vi "Read Enabled Channel Values.vi"(8 "error in (no error)":errorcluster, 11 "Multi Parser in":refnum<class "Multi Sentence Parser.lvclass">) -> (0 "error out":errorcluster, 2 "Enabled Values":dbl[](array[numeric]), 3 "Multi Parser out":refnum<class "Multi Sentence Parser.lvclass">)   [LabVIEW 2024, in "Multi Sentence Parser.lvclass"]
doc: "Multi Sentence Parser.lvclass:Read Enabled Channel Values.vi\n\nThis VI returns the data values of all the channels that are enabled for the Multi Sentence Parser class.\n\nInstrument Communication Module Version 1.0\nOctober, 2018 Original Code Consulting David Thomson\n www.originalcode.com"
uses:
  Multi Sentence Parser.lvclass
  Multi Sentence Parser.lvclass/Multi Sentence Parser.ctl
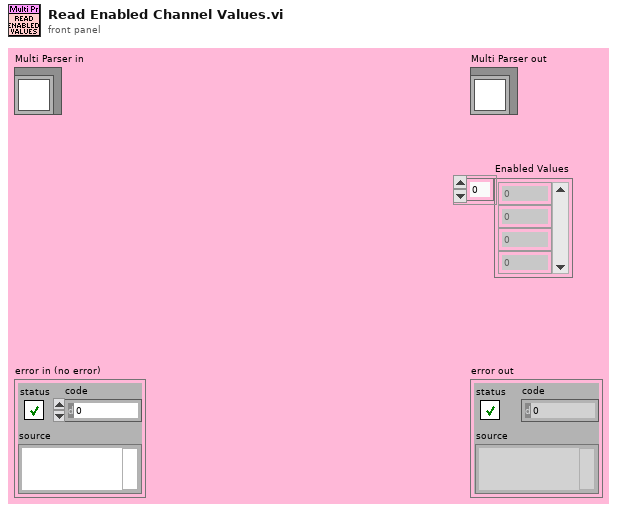
[diagram p1: front panel]
types:
  T1 = cluster{"Sentence ID":string, "Format String":string, "Channels":string[], "Enabled":bool[], "Ignore Missing Sentences?":bool}[]
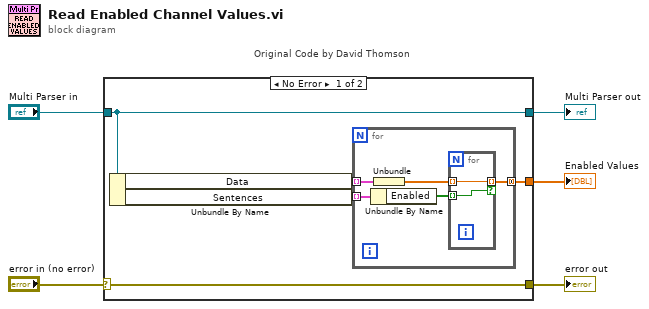
[diagram p0: block diagram]
diagram:
  n1 = case "Original Code by David Thomson" shown="No Error" "error in (no error)" {
    selector: "error in (no error)" -> [w10 w18]
    tunnel: [w10 w18] -> w4
    tunnel: [w8 w19] -> w2
    tunnel: "Multi Parser in" -> [w8 w19]
    tunnel: [w9 _] -> w1
    frame No Error {
      n2 = Unbundle By Name(w8) -> ("Data"=w6:cluster{"1 Sentence":dbl[]}[], "Sentences"=w7:T1)
      n3 = for {
        tunnel: [w14] -> w9 mode=concatenating
        tunnel: w7 -> [w13] mode=indexing
        tunnel: w6 -> [w12] mode=indexing
        n4 = Unbundle By Name(w13) -> ("Enabled"=w15:bool[])
        n5 = Unbundle(w12) -> ("1 Sentence"=w11:dbl[])
        n6 = for {
          tunnel: [w17] -> w14 mode=indexing if=w16
          tunnel: w11 -> [w17] mode=indexing
          tunnel: w15 -> [w16] mode=indexing
        }
      }
    }
    frame Error {
    }
  }
  "error out" <- w4
  "Multi Parser out" <- w2
  "Enabled Values" <- w1
